vi "Page Add.vi"(8 "error in (no error)":errorcluster, 10 "Caption":string, 11 "VI Refnum":refnum<vi>) -> (0 "error out":errorcluster)   [LabVIEW 2018, in "Page.lvlib"]
uses:
  Page.lvlib
  Page Action.ctl
  Page Add.ctl
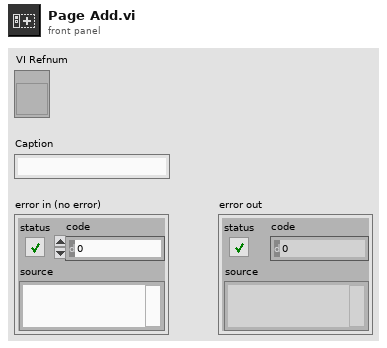
[diagram p1: front panel]
types:
  T1 = typedef "Page.lvlib/Page Add.ctl" = cluster{"VI Path":path, "Caption":string}
  T2 = typedef "Page.lvlib/Page Action.ctl" = enum8{"noop", "new", "init", "close", "page_change", "page_hover", "render", "page_caption", "page_insert", "page_add", "start", "resize", "theme_change", "hide"}
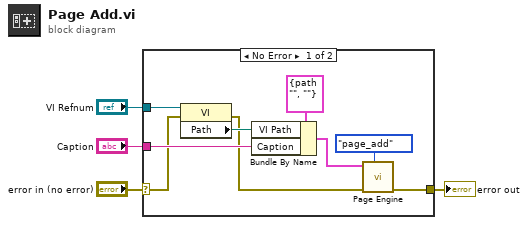
[diagram p0: block diagram]
diagram:
  n1 = case shown="No Error" "error in (no error)" {
    selector: "error in (no error)" -> [w8 w14]
    tunnel: "VI Refnum" -> [w11 _]
    tunnel: "Caption" -> [w9 _]
    tunnel: [w5 w14] -> w1
    frame No Error {
      n2 = property class="VI"(reference=w11, error in=w8) -> (error out=w7:errorcluster, "Path"=w10:path)  [unwired: 1 out]
      n3 = Bundle By Name(cluster=T1 {"VI Path"=path "", "Caption"=""} ("Page Add"), "VI Path"=w10, "Caption"=w9) -> (w6:T1)
      n4 = call "Page Engine.vi"("Action"=Page_Action."page_add", "error in (no error)"=w7, "Data in"=w6) -> ("error out"=w5:errorcluster)  [unwired: 7 in, 1 out]
    }
    frame Error {
    }
  }
  "error out" <- w1
